vi "serpenbot_DDPG_learing_parallel_old_camera_1.vi"() -> ()   [LabVIEW 2020]
uses:
  <vilib>/Analysis/Matrix/Datatypes/RealMatrix.ctl
  <vilib>/Analysis/Matrix/NI_Matrix.lvlib
  <vilib>/Analysis/NI_AALBase.lvlib
  <vilib>/Analysis/baseanly.llb/Real A x B.vi
  <vilib>/Analysis/NI_AALPro.lvlib
  <vilib>/Analysis/Matrix/Numeric/Subtract/Subtract - RM,RM.vi
  <vilib>/Analysis/_algsub.llb/Real PseudoInverse Matrix.vi
panel:
  out "camera_value 2":T1
  out "appended array 3":T1
  out "error out Y":errorcluster
  out "error out X":errorcluster
  out "laser control value":dbl[](array[numeric])
  out "current y":dbl
  out "current x":dbl
  out "control_loop_time":u32
  in  "stop":bool
  in  "Logging":bool caption="Enable"
  in  "k":T1
  in  "Diode Current\nSetting":dbl=3.0
  in  "Laser Repetition\nFrequency":i32=50000
  in  "VISA resource name":refnum<visa-resource-name>="COM14"
  in  "baud rate (9600)":u32=9600
  out "error out":errorcluster
  out "Identification system 1":string
  out "Conn. axes system 1":string[](array[string])
  out "Identification system 2":string
  out "Conn. axes system  2":string[](array[string])
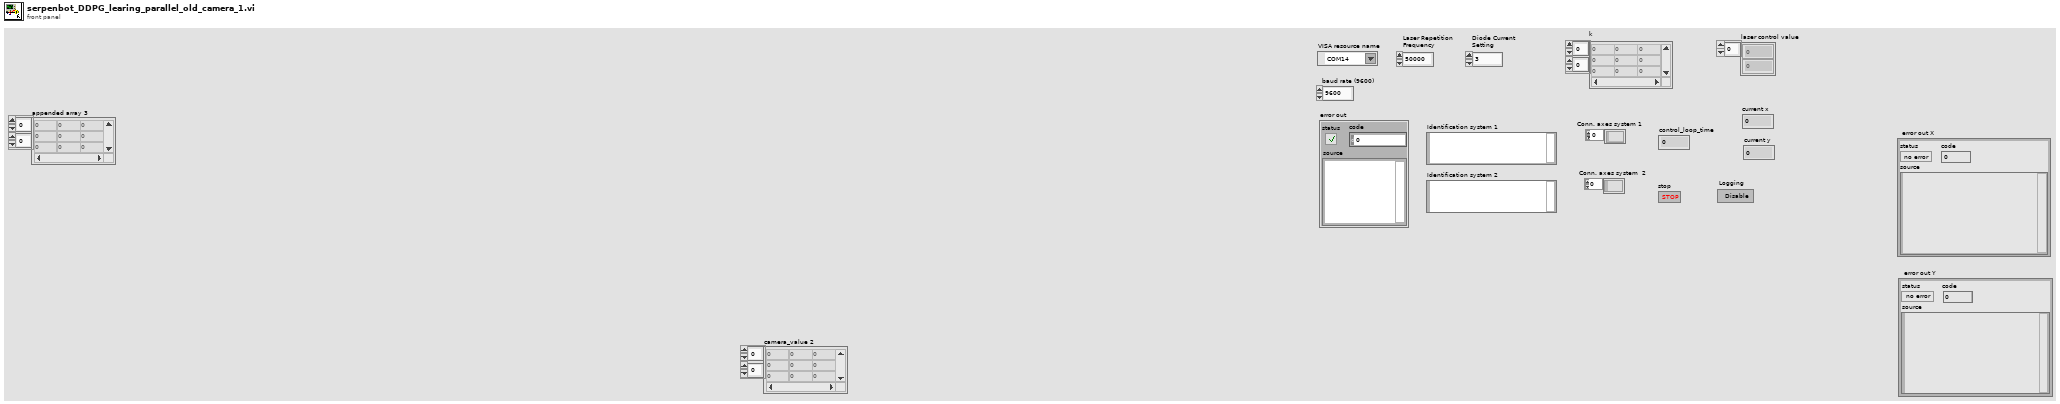
[diagram p1: front panel]
types:
  T1 = typedef "NI_Matrix.lvlib/RealMatrix.ctl" = dbl[][]
  T2 = cluster{"RS232 settings":cluster{"Portnumber":i32, "Baudrate":u16}, "USB settings":cluster{"S/N":string, "USB Search?":bool}, "TCP/IP settings":cluster{"Host address/name":string, "Port":i32, "Board":i32, "TCP/IP Search?":bool}}
  T3 = cluster{"Check FRF?":bool, "Referencing mode":enum16{"FRF (-> FNL)", "FRF", "FNL", "FPL", "RON OFF"}[]}
  T4 = cluster{"Force?":bool, "Dialog?":bool, "Stages":string[]}
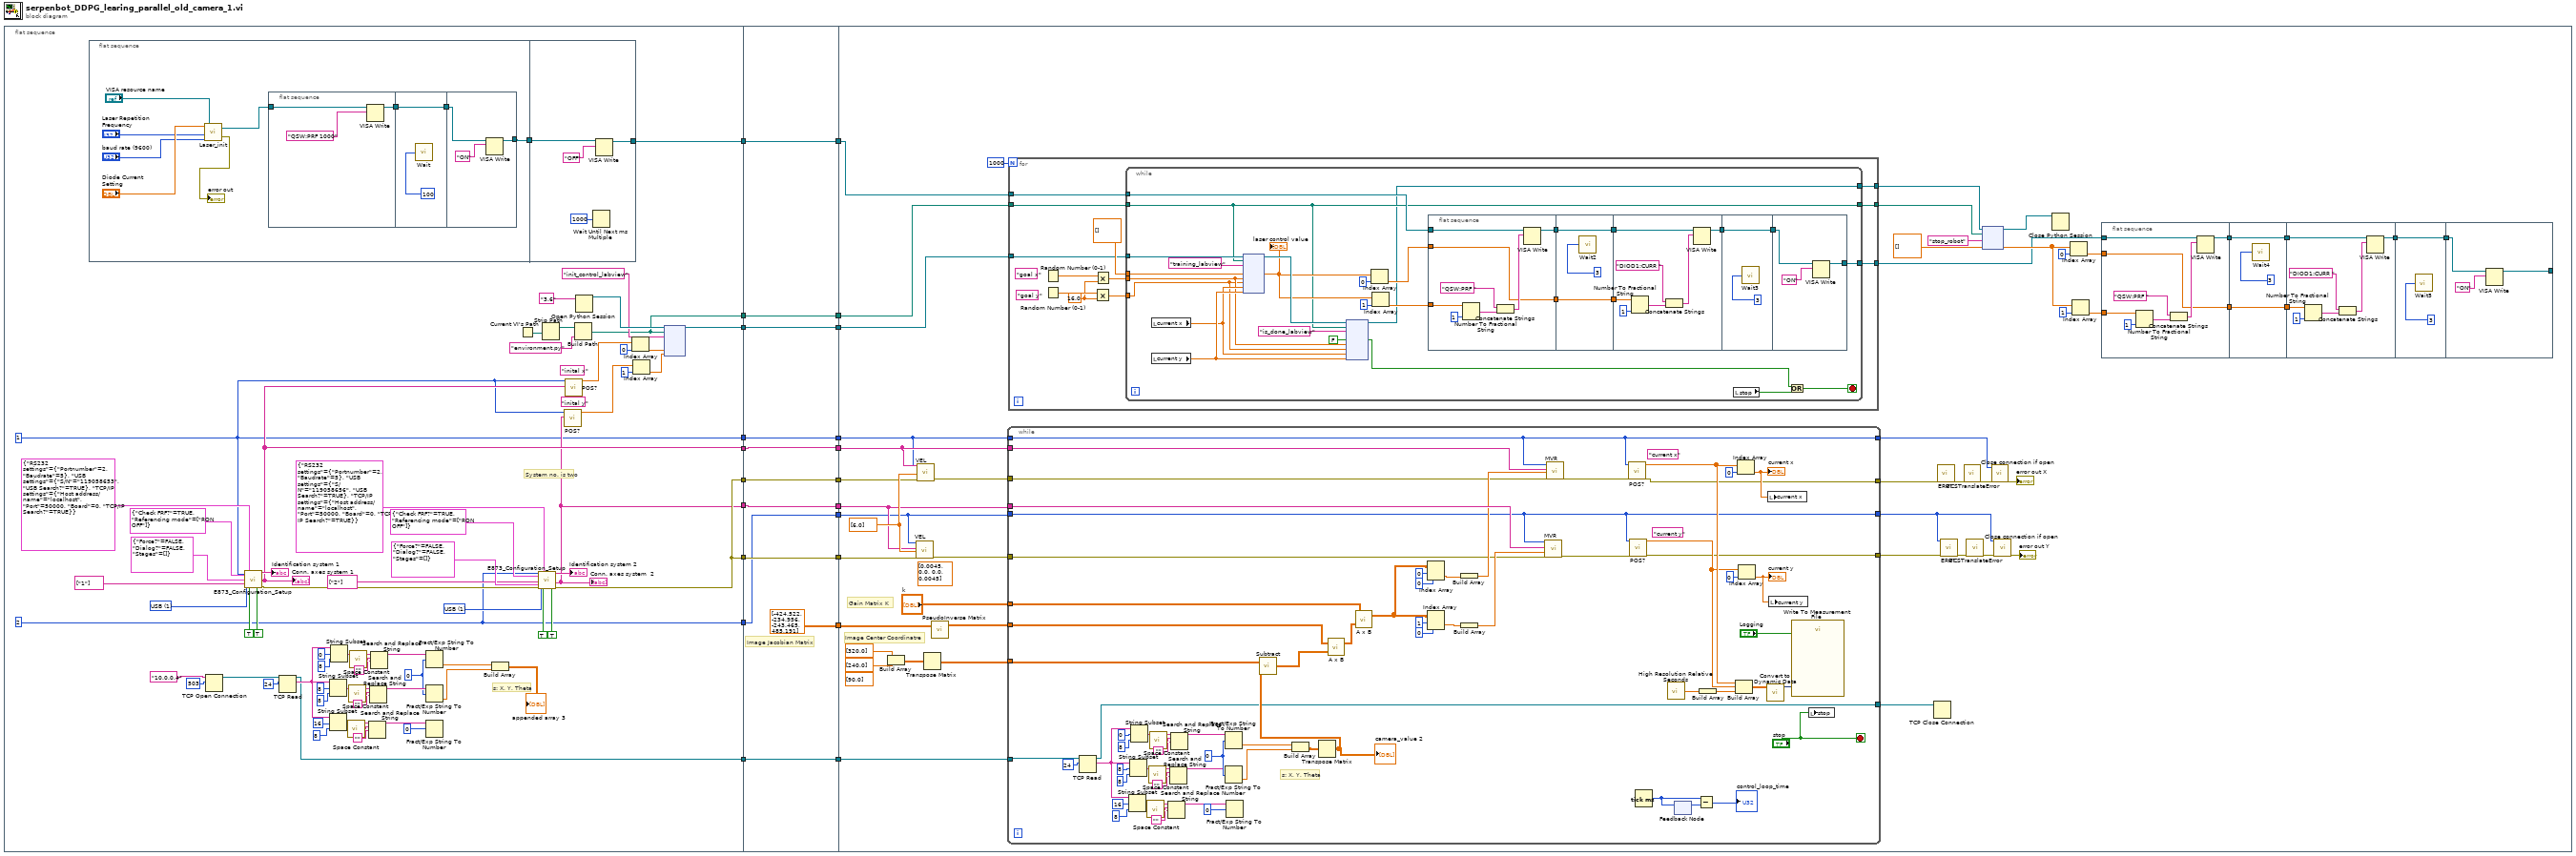
[diagram p0: block diagram]
diagram:
  n1 = flat-sequence {
    tunnel: [w87] -> w21
    tunnel: [w57] -> w20
    tunnel: [w59] -> w19
    tunnel: [w68] -> w18
    tunnel: [w58] -> w17
    tunnel: [w69] -> w16
    tunnel: [w68] -> w15
    tunnel: [w61] -> w14
    tunnel: [w60] -> w13
    tunnel: [w22] -> w2
    tunnel: w21 -> [w120]
    tunnel: [w120] -> w12
    tunnel: w20 -> [w119]
    tunnel: w19 -> [w118]
    tunnel: w18 -> [w117]
    tunnel: w17 -> [w116]
    tunnel: w16 -> [w114]
    tunnel: [w119] -> w11
    tunnel: [w118] -> w10
    tunnel: [w117] -> w9
    tunnel: [w116] -> w8
    tunnel: w15 -> [w115]
    tunnel: [w115] -> w7
    tunnel: [w114] -> w6
    tunnel: [T1 [[-424.522, -234.956], [-243.465, 485.191]] ("J_init 2")] -> w5
    tunnel: w14 -> [w112]
    tunnel: w13 -> [w111]
    tunnel: [w112] -> w4
    tunnel: [w111] -> w3
    tunnel: w2 -> [w110]
    tunnel: [w110] -> w1
    tunnel: w12 -> [w137]
    tunnel: w11 -> [w155]
    tunnel: w10 -> [w162]
    tunnel: w9 -> [w165]
    tunnel: w8 -> [w160]
    tunnel: w7 -> [w164]
    tunnel: w6 -> [w154]
    tunnel: w5 -> [w163]
    tunnel: w4 -> [w139]
    tunnel: w3 -> [w138]
    tunnel: w1 -> [w122]
    frame #0 {
      w36 = 0
      (unwired) "inital y"
      (unwired) "inital x"
      w72 = u16 1 items=["RS232", "USB", "TCP/IP"] ("Interface")
      w75 = u16 1 items=["RS232", "USB", "TCP/IP"] ("Interface")
      w69 = 2 ("System no.")
      w57 = 1 ("System no.")
      # "s: X, Y, Theta"
      # "System no. is two"
      n2 = flat-sequence {
        tunnel: [w89] -> w88
        tunnel: w88 -> [w107]
        tunnel: [w106] -> w87
        frame #0 {
          n3 = call "Laser_init.vi"("baud rate (9600)"="baud rate (9600)", "Laser Repetition\nFrequency"="Laser Repetition\nFrequency", "VISA resource name"="VISA resource name", "Diode Current\nSetting"="Diode Current\nSetting") -> ("error out"=→"error out":errorcluster, "VISA Refnum out"=w90:refnum<visa-resource-name>)
          n4 = flat-sequence {
            tunnel: w90 -> [w100]
            tunnel: [w99] -> w97
            tunnel: w97 -> [w102]
            tunnel: [w102] -> w96
            tunnel: w96 -> [w103]
            tunnel: [w104] -> w89
            frame #0 {
              n5 = VISA Write(VISA resource name=w100, write buffer="QSW:PRF 1000" ("string")) -> (VISA resource name out=w99:refnum<visa-resource-name>)  [unwired: 1 in, 2 out]
            }
            frame #1 {
              n6 = call "Wait"("Count(mSec)"=u32 100) -> ()  [unwired: 1 out]
            }
            frame #2 {
              n7 = VISA Write(VISA resource name=w103, write buffer="ON") -> (VISA resource name out=w104:refnum<visa-resource-name>)  [unwired: 1 in, 2 out]
            }
          }
        }
        frame #1 {
          n8 = Wait Until Next ms Multiple(millisecond multiple=u32 1000) -> ()  [unwired: 1 out]
          n9 = VISA Write(VISA resource name=w107, write buffer="OFF") -> (VISA resource name out=w106:refnum<visa-resource-name>)  [unwired: 1 in, 2 out]
        }
      }
      n10 = TCP Open Connection(address="10.0.0.4", remote port or service name=u16 503) -> (connection ID=w46:refnum<k5>)  [unwired: 3 in, 1 out]
      n11 = call "E873_Configuration_Setup.vi"("System no."=w57, "Referencing"=T3 {"Check FRF?"=TRUE, "Referencing mode"=[enum."RON OFF"]}, "Interface"=w75, "All axes?"=TRUE, "Axes to move"=string[] ["1"], "Interface settings"=T2 {"RS232 settings"={"Portnumber"=2, "Baudrate"=5}, "USB settings"={"S/N"="119058653", "USB Search?"=TRUE}, "TCP/IP settings"={"Host address/name"="localhost", "Port"=50000, "Board"=0, "TCP/IP Search?"=TRUE}}, "Stage selection"=T4 {"Force?"=FALSE, "Dialog?"=FALSE, "Stages"=[]}, "Switch servo on?"=TRUE ("Use dialog to define\nconnected stages?")) -> ("Identification"=→"Identification system 1":string, "Conn. \nAxes"=w59:string[], "error out"=w84:errorcluster)  [unwired: 4 in, 5 out]
      "Conn. axes system 1" <- w59
      n12 = TCP Read(connection ID=w46, bytes to read=24) -> (connection ID out=w22:refnum<k5>, data out=w45:string)  [unwired: 3 in, 1 out]
      n13 = String Subset(string=w45, offset (0)=16, length (rest)=8 ("length (rest)")) -> (substring=w43:string)
      n14 = String Subset(string=w45, offset (0)=8, length (rest)=8 ("length (rest)")) -> (substring=w44:string)
      n15 = String Subset(string=w45, offset (0)=0, length (rest)=8 ("length (rest)")) -> (substring=w42:string)
      n16 = call <vilib>:"Space Constant.vi"() -> ("String"=w41:string)
      n17 = call <vilib>:"Space Constant.vi"() -> ("String"=w40:string)
      n18 = call <vilib>:"Space Constant.vi"() -> ("String"=w39:string)
      n19 = Search and Replace String(input string=w43, search string=w41, replace string="") -> (result string=w47:string)  [unwired: 5 in, 3 out]
      n20 = Search and Replace String(input string=w44, search string=w40, replace string="") -> (result string=w48:string)  [unwired: 5 in, 3 out]
      n21 = Search and Replace String(input string=w42, search string=w39, replace string="") -> (result string=w49:string)  [unwired: 5 in, 3 out]
      n22 = Fract/Exp String To Number(string=w49, offset=w36) -> (number=w37:dbl)  [unwired: 2 in, 1 out]
      n23 = Fract/Exp String To Number(string=w48, offset=w36) -> (number=w38:dbl)  [unwired: 2 in, 1 out]
      n24 = Fract/Exp String To Number(string=w47, offset=0) -> ()  [unwired: 2 in, 2 out]
      n25 = Build Array(w37, w38) -> (→"appended array 3":T1)
      n26 = Current VI's Path() -> (path=w67:path)
      n27 = call "E873_Configuration_Setup.vi"("System no."=w69, "Referencing"=T3 {"Check FRF?"=TRUE, "Referencing mode"=[enum."RON OFF"]}, "Interface"=w72, "All axes?"=TRUE, "Axes to move"=string[] ["2"], "error in"=w84, "Interface settings"=T2 {"RS232 settings"={"Portnumber"=2, "Baudrate"=5}, "USB settings"={"S/N"="119058656", "USB Search?"=TRUE}, "TCP/IP settings"={"Host address/name"="localhost", "Port"=50000, "Board"=0, "TCP/IP Search?"=TRUE}}, "Stage selection"=T4 {"Force?"=FALSE, "Dialog?"=FALSE, "Stages"=[]}, "Switch servo on?"=TRUE ("Use dialog to define\nconnected stages?")) -> ("Identification"=→"Identification system 2":string, "Conn. \nAxes"=w58:string[], "error out"=w68:errorcluster)  [unwired: 3 in, 5 out]
      "Conn. axes system  2" <- w58
      n28 = Strip Path(path=w67) -> (stripped path=w66:path)  [unwired: 1 out]
      n29 = call "POS?.vi"("System no."=w57, "Axes to query"=w58) -> ("Position"=w51:dbl[])  [unwired: 3 in, 14 out]
      n30 = call "POS?.vi"("System no."=w57, "Axes to query"=w59) -> ("Position"=w54:dbl[])  [unwired: 3 in, 14 out]
      n31 = Build Path(base path=w66, name or relative path="environment.py") -> (appended path=w61:path)
      n32 = Open Python Session(python version="3.6" ("Python version")) -> (session out=w63:refnum<k35>)  [unwired: 2 in, 1 out]
      n33 = Index Array(array=w54, index=0) -> (element=w55:dbl)
      n34 = Index Array(array=w51, index=1) -> (element=w52:dbl)
      n35 = node(w63, w61, "init_control_labview" ("function name"), w55, w52) -> (w60:refnum<k35>)  [unwired: 5 in, 3 out]
    }
    frame #1 {
      # "Image Jacobian Matrix"
    }
    frame #2 {
      w166 = dbl[] [6.0] ("Velocity values")
      (unwired) T1 [[0.0045, 0.0], [0.0, 0.0045]] ("J_init 2")
      (unwired) dbl[] [90.0] ("element")
      # "Gain Matrix K"
      # "Image Center Coordinatre"
      n36 = Build Array(dbl[] [320.0] ("element"), dbl[] [240.0] ("element")) -> (w167:T1)
      n37 = call "VEL.vi"("System no."=w154, "Axes to set"=w160, "Velocity values"=w166, "error in"=w164) -> ("error out"=w159:errorcluster)  [unwired: 2 in, 13 out]
      n38 = call "VEL.vi"("System no."=w155, "Axes to set"=w162, "Velocity values"=w166, "error in"=w165) -> ("error out"=w161:errorcluster)  [unwired: 2 in, 13 out]
      n39 = Transpose Matrix(1:w167) -> (0:w156:T1)
      n40 = call-poly <vilib>:"PseudoInverse Matrix.vi"("Input Matrix"=w163) -> ("PseudoInverse Matrix"=w157:T1)  [unwired: 1 in, 1 out]
      n41 = while {
        tunnel: w159 -> [w281]
        tunnel: w154 -> [w262]
        tunnel: w160 -> [w299]
        tunnel: w161 -> [w282]
        tunnel: w162 -> [w298]
        tunnel: w155 -> [w264]
        tunnel: w157 -> [w287]
        tunnel: "k" -> [w286]
        tunnel: w156 -> [w285]
        tunnel: [w264] -> w126
        tunnel: [w263] -> w125
        tunnel: [w262] -> w124
        tunnel: [w261] -> w123
        tunnel: w122 -> [w234]
        tunnel: [w233] -> w121
        stop <- "stop" stop-if-true
        w260 = 0
        (unwired) "current y"
        (unwired) "current x"
        # "s: X, Y, Theta"
        n42 = TCP Read(connection ID=w234, bytes to read=24) -> (connection ID out=w233:refnum<k5>, data out=w241:string)  [unwired: 3 in, 1 out]
        n43 = String Subset(string=w241, offset (0)=16, length (rest)=8 ("length (rest)")) -> (substring=w243:string)
        n44 = String Subset(string=w241, offset (0)=8, length (rest)=8 ("length (rest)")) -> (substring=w242:string)
        n45 = String Subset(string=w241, offset (0)=0, length (rest)=8 ("length (rest)")) -> (substring=w248:string)
        n46 = call <vilib>:"Space Constant.vi"() -> ("String"=w251:string)
        n47 = call <vilib>:"Space Constant.vi"() -> ("String"=w253:string)
        n48 = call <vilib>:"Space Constant.vi"() -> ("String"=w255:string)
        n49 = Search and Replace String(input string=w243, search string=w251, replace string="") -> (result string=w239:string)  [unwired: 5 in, 3 out]
        n50 = Search and Replace String(input string=w242, search string=w253, replace string="") -> (result string=w238:string)  [unwired: 5 in, 3 out]
        n51 = Search and Replace String(input string=w248, search string=w255, replace string="") -> (result string=w237:string)  [unwired: 5 in, 3 out]
        n52 = Fract/Exp String To Number(string=w237, offset=w260) -> (number=w259:dbl)  [unwired: 2 in, 1 out]
        n53 = Fract/Exp String To Number(string=w238, offset=w260) -> (number=w258:dbl)  [unwired: 2 in, 1 out]
        n54 = Fract/Exp String To Number(string=w239, offset=0) -> ()  [unwired: 2 in, 2 out]
        n55 = Build Array(w259, w258) -> (w236:T1)
        n56 = Transpose Matrix(1:w236) -> (0:w235:T1)
        "camera_value 2" <- w235
        n57 = call-poly <vilib>:"Subtract.vi"("Real Matrix B"=w235, "Real Matrix A"=w285) -> ("A - B"=w293:T1)
        n58 = call-poly <vilib>:"A x B.vi"("B"=w293, "A"=w287) -> ("A x B"=w291:T1)  [unwired: 1 out]
        n59 = call-poly <vilib>:"A x B.vi"("B"=w291, "A"=w286) -> ("A x B"=w292:T1)  [unwired: 1 out]
        n60 = Index Array(array=w292, index (row)=0, index (col)=0) -> (element=w284:dbl)
        n61 = Index Array(array=w292, index (row)=1, index (col)=0) -> (element=w283:dbl)
        n62 = Build Array(w284) -> (w290:dbl[])
        n63 = Build Array(w283) -> (w289:dbl[])
        n64 = call "MVR.vi"("System no."=w262, "Axes to move"=w299, "Position values"=w289, "error in"=w281) -> ("error out"=w273:errorcluster)  [unwired: 1 in, 14 out]
        n65 = call "MVR.vi"("System no."=w264, "Axes to move"=w298, "Position values"=w290, "error in"=w282) -> ("error out"=w274:errorcluster)  [unwired: 1 in, 14 out]
        n66 = call "POS?.vi"("System no."=w264, "error in"=w274) -> ("Position"=w271:dbl[], "error out"=w263:errorcluster)  [unwired: 3 in, 13 out]
        n67 = call "POS?.vi"("System no."=w262, "error in"=w273) -> ("Position"=w269:dbl[], "error out"=w261:errorcluster)  [unwired: 3 in, 13 out]
        n68 = Tick Count (ms)() -> (millisecond timer value=w272:u32)
        n69 = call <vilib>:"High Resolution Relative Seconds.vi"() -> ("relative seconds"=w276:dbl)
        n70 = feedback #1() -> (w288:u32)  [unwired: 1 in]
        n71 = feedback-in #1(w272) -> ()
        n72 = Subtract(x=w272, y=w288) -> (x-y=→"control_loop_time":u32)
        n73 = Build Array(w276) -> (w275:dbl[])
        n74 = Build Array(w271, w269, w275) -> (w278:dbl[][])
        n75 = Index Array(array=w271, index=0) -> (element=w267:dbl)
        "current x" <- w267
        n76 = Index Array(array=w269, index=0) -> (element=w266:dbl)
        "current y" <- w266
        n77 = call "Convert to Dynamic Data"("2D Array"=w278) -> ("Dynamic Data Type"=w277:dynamicdata)  [unwired: 3 in]
        n78 = local write "current x"(w267) -> ()
        n79 = local write "current y"(w266) -> ()
        n80 = call "Write To Measurement File"("Signals"=w277, "Enable"="Logging") -> ()  [unwired: 15 in, 3 out]
        n81 = local write "stop"("stop") -> ()
      }
      n82 = for {
        N: 1000 -> [_]
        tunnel: w139 -> [w175]
        tunnel: w138 -> [w174]
        tunnel: w137 -> [w173]
        tunnel: [w172] -> w135
        tunnel: [w171] -> w134
        tunnel: [w170] -> w133
        w179 = 16.0
        (unwired) "goal y"
        (unwired) "goal x"
        n83 = Random Number (0-1)() -> (number: 0 to 1=w181:dbl)
        n84 = Random Number (0-1)() -> (number: 0 to 1=w180:dbl)
        n85 = Multiply(x=w180, y=w179) -> (x*y=w176:dbl)
        n86 = Multiply(x=w181, y=w179) -> (x*y=w177:dbl)
        n87 = while {
          tunnel: dbl[] [] -> [w194]
          tunnel: w177 -> [w191]
          tunnel: w176 -> [w190]
          tunnel: w175 -> [w187]
          tunnel: w174 -> [w189]
          tunnel: w173 -> [w188]
          tunnel: [w187] -> w172
          tunnel: [w186] -> w171
          tunnel: [w183] -> w170
          stop <- w184 stop-if-true
          n88 = local read "current x"() -> (w192:dbl)
          n89 = local read "current y"() -> (w193:dbl)
          n90 = node(w189, w187, "training_labview" ("function name"), w194, w191, w190, w192, w193) -> (w202:refnum<k35>, w196:dbl[])  [unwired: 5 in, 3 out]
          "laser control value" <- w196
          n91 = node(w202, w187, "is_done_labview" ("function name"), FALSE, w191, w190, w192, w193) -> (w186:refnum<k35>, w182:bool)  [unwired: 5 in, 3 out]
          n92 = Index Array(array=w196, index=0) -> (element=w199:dbl)
          n93 = Index Array(array=w196, index=1) -> (element=w195:dbl)
          n94 = flat-sequence {
            tunnel: w188 -> [w213]
            tunnel: [w212] -> w209
            tunnel: w195 -> [w211]
            tunnel: w199 -> [w210]
            tunnel: [w210] -> w208
            tunnel: [w220] -> w207
            tunnel: [w218] -> w206
            tunnel: w209 -> [w220]
            tunnel: w208 -> [w218]
            tunnel: [w227] -> w205
            tunnel: w207 -> [w225]
            tunnel: w206 -> [w222]
            tunnel: w205 -> [w229]
            tunnel: [w229] -> w204
            tunnel: w204 -> [w231]
            tunnel: [w230] -> w183
            frame #0 {
              n95 = Number To Fractional String(number=w211, precision (6)=i16 1) -> (F-format string=w216:string)  [unwired: 2 in]
              n96 = Concatenate Strings("QSW:PRF " ("string"), w216) -> (w217:string)
              n97 = VISA Write(VISA resource name=w213, write buffer=w217) -> (VISA resource name out=w212:refnum<visa-resource-name>)  [unwired: 1 in, 2 out]
            }
            frame #1 {
              n98 = call "Wait2"("Count(mSec)"=u32 3) -> ()  [unwired: 1 out]
            }
            frame #2 {
              n99 = Number To Fractional String(number=w222, precision (6)=i16 1) -> (F-format string=w223:string)  [unwired: 2 in]
              n100 = Concatenate Strings("DIOD1:CURR " ("string"), w223) -> (w226:string)
              n101 = VISA Write(VISA resource name=w225, write buffer=w226) -> (VISA resource name out=w227:refnum<visa-resource-name>)  [unwired: 1 in, 2 out]
            }
            frame #3 {
              n102 = call "Wait3"("Count(mSec)"=u32 3) -> ()  [unwired: 1 out]
            }
            frame #4 {
              n103 = VISA Write(VISA resource name=w231, write buffer="ON") -> (VISA resource name out=w230:refnum<visa-resource-name>)  [unwired: 1 in, 2 out]
            }
          }
          n104 = local read "stop"() -> (w185:bool)
          n105 = Or(x=w182, y=w185) -> (x .or. y?=w184:bool)
        }
      }
      n106 = TCP Close Connection(connection ID=w121) -> ()  [unwired: 2 in, 2 out]
      n107 = call "ERR?.vi"("error in"=w125) -> ("error out"=w130:errorcluster)  [unwired: 1 in, 17 out]
      n108 = call "ERR?.vi"("System no."=w124, "error in"=w123) -> ("error out"=w127:errorcluster)  [unwired: 17 out]
      n109 = call "GCSTranslateError.vi"("error in"=w130) -> ("error out"=w131:errorcluster)  [unwired: 18 out]
      n110 = call "GCSTranslateError.vi"("error in"=w127) -> ("error out"=w128:errorcluster)  [unwired: 18 out]
      n111 = node(w134, w135, "stop_robot" ("function name"), dbl[] []) -> (w145:refnum<k35>, w140:dbl[])  [unwired: 1 in, 3 out]
      n112 = call "Close connection if open.vi"("System no."=w126, "error in"=w131) -> ("error out"=→"error out X":errorcluster)  [unwired: 1 in, 16 out]
      n113 = call "Close connection if open.vi"("System no."=w124, "error in"=w128) -> ("error out"=→"error out Y":errorcluster)  [unwired: 1 in, 16 out]
      n114 = Close Python Session(session in=w145) -> ()  [unwired: 1 in, 1 out]
      n115 = Index Array(array=w140, index=0) -> (element=w142:dbl)
      n116 = Index Array(array=w140, index=1) -> (element=w141:dbl)
      n117 = flat-sequence {
        tunnel: w133 -> [w303]
        tunnel: [w302] -> w153
        tunnel: w141 -> [w301]
        tunnel: w142 -> [w300]
        tunnel: [w300] -> w152
        tunnel: [w310] -> w151
        tunnel: [w308] -> w150
        tunnel: w153 -> [w310]
        tunnel: w152 -> [w308]
        tunnel: [w317] -> w149
        tunnel: w151 -> [w315]
        tunnel: w150 -> [w312]
        tunnel: w149 -> [w319]
        tunnel: [w319] -> w148
        tunnel: w148 -> [w321]
        tunnel: [w320] -> _
        frame #0 {
          n118 = Number To Fractional String(number=w301, precision (6)=i16 1) -> (F-format string=w306:string)  [unwired: 2 in]
          n119 = Concatenate Strings("QSW:PRF " ("string"), w306) -> (w307:string)
          n120 = VISA Write(VISA resource name=w303, write buffer=w307) -> (VISA resource name out=w302:refnum<visa-resource-name>)  [unwired: 1 in, 2 out]
        }
        frame #1 {
          n121 = call "Wait4"("Count(mSec)"=u32 3) -> ()  [unwired: 1 out]
        }
        frame #2 {
          n122 = Number To Fractional String(number=w312, precision (6)=i16 1) -> (F-format string=w313:string)  [unwired: 2 in]
          n123 = Concatenate Strings("DIOD1:CURR " ("string"), w313) -> (w316:string)
          n124 = VISA Write(VISA resource name=w315, write buffer=w316) -> (VISA resource name out=w317:refnum<visa-resource-name>)  [unwired: 1 in, 2 out]
        }
        frame #3 {
          n125 = call "Wait5"("Count(mSec)"=u32 3) -> ()  [unwired: 1 out]
        }
        frame #4 {
          n126 = VISA Write(VISA resource name=w321, write buffer="ON") -> (VISA resource name out=w320:refnum<visa-resource-name>)  [unwired: 1 in, 2 out]
        }
      }
    }
  }
